vi "Update Results.vi"(0 "IMeasurementService in":refnum<class "IMeasurementService.lvclass">, 5 "Measurement Results":variant, 7 "MeasurementPluginService in":refnum<class "MeasurementPluginService.lvclass">, 9 "gRPCid in":T1, 11 "error in (no error)":errorcluster) -> (4 "IMeasurementService out":refnum<class "IMeasurementService.lvclass">, 8 "MeasurementPluginService out":refnum<class "MeasurementPluginService.lvclass">, 15 "error out":errorcluster)   [LabVIEW 2020, in "MeasurementLink Measurement Server.lvlib" / "IMeasurementService.lvclass"]
uses:
  IMeasurementService.lvclass
  <vilib>/gRPC/LabVIEW gRPC Library/Shared/grpcId.ctl
  MeasurementPluginService/MeasurementPluginService.lvclass
  <vilib>/gRPC/LabVIEW gRPC Library/grpc-lvsupport-release.lvlib
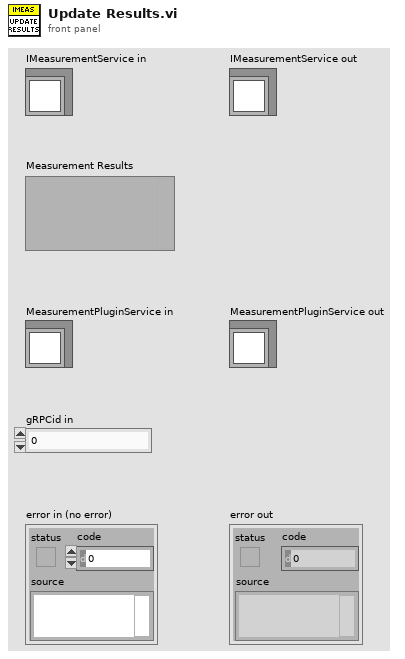
[diagram p1: front panel]
types:
  T1 = typedef "grpc-lvsupport-release.lvlib/grpcId.ctl" = u64
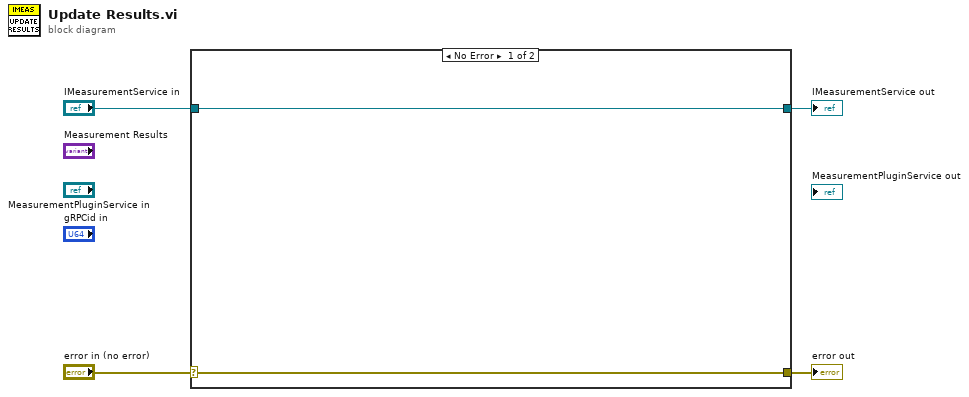
[diagram p0: block diagram]
diagram:
  n1 = case shown="No Error" "error in (no error)" {
    selector: "error in (no error)" -> [w5 w8]
    tunnel: [w5 w8] -> w3
    tunnel: [w6 w7] -> w1
    tunnel: "IMeasurementService in" -> [w6 w7]
    frame No Error {
    }
    frame Error {
    }
  }
  "error out" <- w3
  "IMeasurementService out" <- w1
